vi "FTW-JSON-ToLabVIEW.vi"(0 "Type and Defaults":variant, 5 "JSON String":string, 11 "error in":errorcluster) -> (4 "Populated Values":variant, 15 "error out":errorcluster)   [LabVIEW 2012]
uses:
  Regex/FTW-Regex.vi
  FTW-JSON-RegexHeader.vi
  Error/FTW-ERR-ThrowError.vi
  Container/FTW-Container.lvclass
panel:
  # "Inputs"
  # "Outputs"
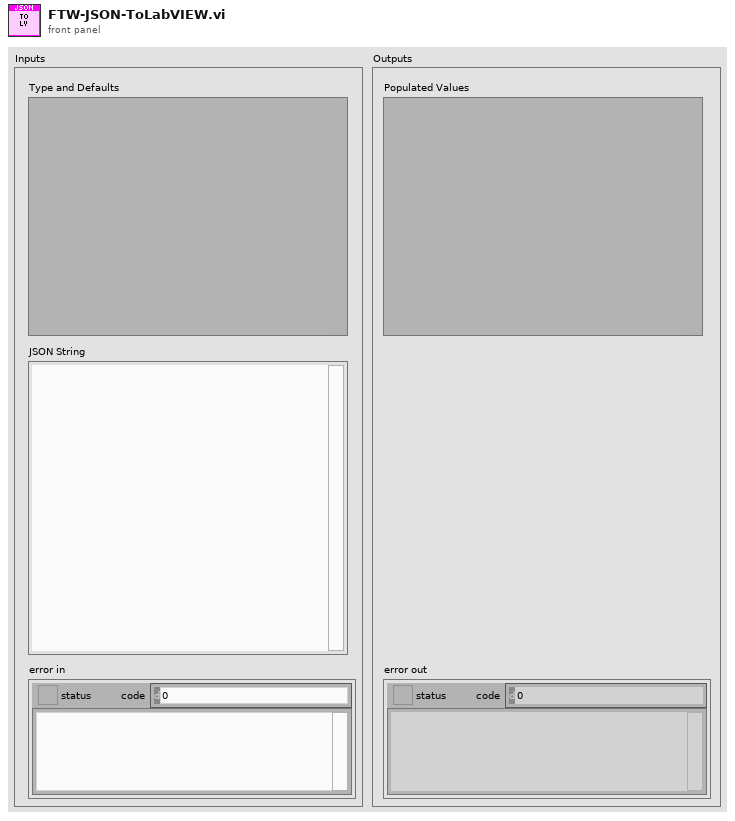
[diagram p1: front panel]
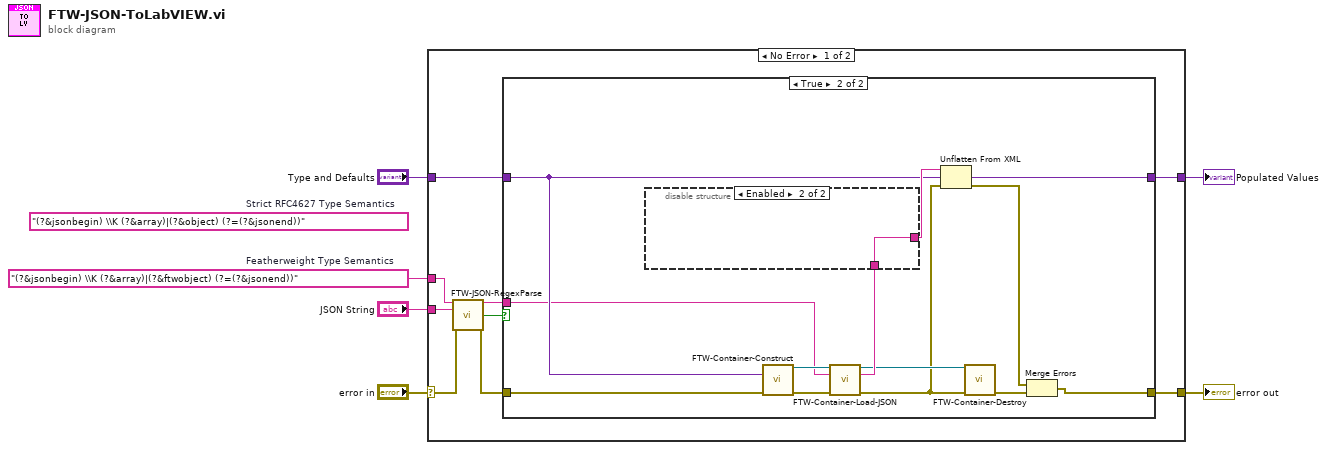
[diagram p0: block diagram]
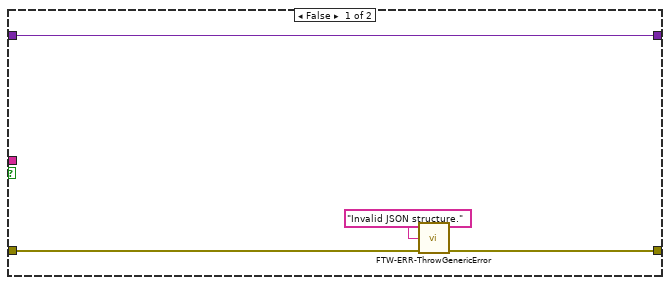
[diagram p2: hidden frame]
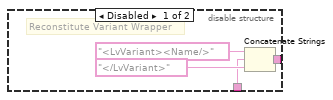
[diagram p3: hidden frame]
diagram:
  (unwired) "(?&jsonbegin) \\K (?&array)|(?&object) (?=(?&jsonend))"  # Strict RFC4627 Type Semantics
  w1 = "(?&jsonbegin) \\K (?&array)|(?&ftwobject) (?=(?&jsonend))"  # Featherweight Type Semantics
  n1 = case shown="No Error" "error in" {
    selector: "error in" -> [w9 w38]
    tunnel: "JSON String" -> [w15 _]
    tunnel: "Type and Defaults" -> [w14 w39]
    tunnel: [w13 w39] -> w4
    tunnel: [w10 w38] -> w3
    tunnel: w1 -> [w7 _]
    frame No Error {
      n2 = call "FTW-JSON-RegexParse.vi"("Regular Expression using JSON subroutines"=w7, "Input String"=w15, "error in"=w9) -> ("Match"=w12:string, "Found Match?"=w8:bool, "error out"=w11:errorcluster)  [unwired: 8 in, 2 out]
      n3 = case shown="True" w8 {
        tunnel: w14 -> [w16 w28]
        tunnel: [w16 w32] -> w13
        tunnel: w12 -> [_ w25]
        tunnel: w11 -> [w19 w27]
        tunnel: [w18 w29] -> w10
        frame False {
          n4 = call "FTW-ERR-ThrowGenericError.vi"("Error Message"="Invalid JSON structure.", "error in"=w19) -> ("error out"=w18:errorcluster)  [unwired: 13 in]
        }
        frame True {
          n5 = call "FTW-Container-Construct.vi"("LabVIEW Data Structure"=w28, "error in"=w27) -> ("Container"=w26:refnum<class "FTW-Container.lvclass">, "error out"=w22:errorcluster)  [unwired: 12 in]
          n6 = call "FTW-Container-Load-JSON.vi"("Container"=w26, "JSON to Load"=w25, "error in"=w22) -> ("Container out"=w23:refnum<class "FTW-Container.lvclass">, "Serialized Node"=w24:string, "error out"=w20:errorcluster)  [unwired: 10 in]
          n7 = disable-structure shown="Enabled" {
            disable-tunnel: [w35 w37] -> w31
            disable-tunnel: w24 -> [w33 w37]
            frame Disabled {
              # "Reconstitute Variant Wrapper"
              n8 = Concatenate Strings("<LvVariant><Name/>" ("string"), w33, "</LvVariant>" ("string")) -> (w35:string)
            }
            frame Enabled {
            }
          }
          n9 = Unflatten From XML(xml string=w31, type=w28, error in (no error)=w20) -> (value=w32:variant, error out=w30:errorcluster)
          n10 = call "FTW-Container-Destroy.vi"("Container"=w23, "error in"=w20) -> ("error out"=w21:errorcluster)  [unwired: 13 in]
          n11 = Merge Errors(w30, w21) -> (w29:errorcluster)
        }
      }
    }
    frame Error {
    }
  }
  "error out" <- w3
  "Populated Values" <- w4
